vi "Write Guests History Data.vi"(0 "Guest History Map":map{string, T1}(c390), 11 "error in (no error)":errorcluster) -> (15 "error out":errorcluster)   [LabVIEW 2023, in "File Data Manager.lvlib" / "File Data Manager.lvclass"]
uses:
  File Data Manager.lvclass
  Central Data Manager/Central Data Manager/Guest Details.ctl
  <vilib>/Utility/file.llb/Write Delimited Spreadsheet (string).vi
  File Data Manager.lvclass/File Data Manager.ctl
  Utilities/Utilities.lvlib
  Central Data Manager/Central Data Manager/Central Data Manager.lvclass
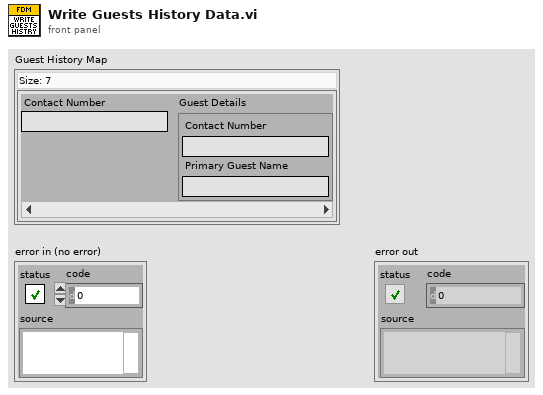
[diagram p1: front panel]
types:
  T1 = typedef "Central Data Manager.lvlib/Central Data Manager.lvclass/Guest Details.ctl" = cluster{"Contact Number":string, "Primary Guest Name":string}
  T2 = typedef "Hotel Management Tool Model.lvlib/Hotel Management Tool Model.lvclass/Database File Paths.ctl" = cluster{"Food Menu File Path":path, "Guests Histroy File Path":path, "Room Size File Path":path, "Rooms List File Path":path, "Rooms Service Allocation File Path":path, "Staff List File Path":path}
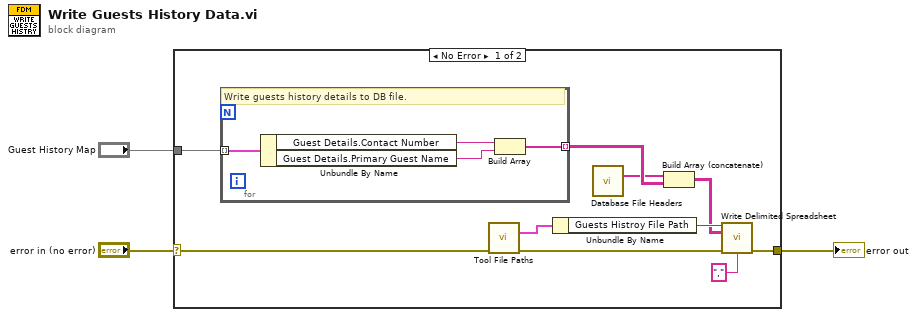
[diagram p0: block diagram]
diagram:
  n1 = case shown="No Error" "error in (no error)" {
    selector: "error in (no error)" -> [w11 w18]
    tunnel: [w8 w18] -> w1
    tunnel: "Guest History Map" -> [w10 _]
    frame No Error {
      n2 = for {
        tunnel: w10 -> [w17] mode=indexing
        tunnel: [w15] -> w9 mode=indexing
        # "Write guests history details to DB file."
        n3 = Unbundle By Name(w17) -> ("Guest Details.Contact Number"=w14:string, "Guest Details.Primary Guest Name"=w16:string)
        n4 = Build Array(w14, w16) -> (w15:string[])
      }
      n5 = call "Tool File Paths.vi"("error in (no error)"=w11) -> ("Database File Paths"=w13:T2, "error out"=w12:errorcluster)  [unwired: 12 in, 1 out]
      n6 = Unbundle By Name(w13) -> ("Guests Histroy File Path"=w7:path)
      n7 = call "Database File Headers.vi"() -> ("Guests History Headers"=w4:string[])  [unwired: 13 in, 2 out]
      n8 = Build Array (concatenate)(w4, w9) -> (w5:string[][])
      n9 = call-poly <vilib>:"Write Delimited Spreadsheet.vi"("file path (dialog if empty)"=w7, "2D data"=w5, "error in (no error)"=w12, "delimiter (\\t)"="," ("delimiter (\\t)")) -> ("error out"=w8:errorcluster)  [unwired: 10 in, 1 out]
    }
    frame Error {
    }
  }
  "error out" <- w1
